vi "Intake.vi"(10 "Enum":enum16{"Retract", "Extend"}(ring)) -> ()   [LabVIEW 2019]
uses:
  <vilib>/Rock Robotics/WPI/ThirdParty/Phoenix-LabVIEW/Motor Controller/Controls/CTRE_Phoenix_MotorControl_ControlMode.ctl
  <vilib>/Rock Robotics/WPI/Solenoid/WPI_SolenoidValue.ctl
  max2020/RoboRIO/Global Data.vi
  max2020/RoboRIO/Refnums.vi
  <vilib>/Rock Robotics/WPI/Solenoid/WPI_SolenoidSetEnum.vi
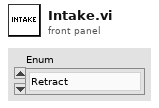
[diagram p1: front panel]
types:
  T1 = typedef "CTRE_Phoenix_MotorControl_ControlMode.ctl" = u16
  T2 = typedef "WPI_RobotDriveDevRef.ctl" = cluster{"DevStatus":errorcluster, "Motors[]":T3[], "Square Inputs":bool, "Max Output":dbl}
  T3 = typedef "WPI_MotorControlDeviceRef.ctl" = cluster{"DeviceStatus":errorcluster, "Type":T4, "PWM":cluster{"PWM Channel":T5, "DeadBand":T6}, "CAN":cluster{"Device Number":u8, "SetOutput VI Ref":variant, "GetOutput VI Ref":variant, "Enable VI Ref":variant, "Disable VI Ref":variant, "Data":variant}, "Invert":bool, "DIO PWM":cluster{"PWM \"Enable\" Channel":T5, "DIOChannel":T7, "PWM Rate":dbl}}
  T4 = typedef "WPI_MotorControlType.ctl" = enum16{"PWM", "CAN", "DIO PWM"}
  T5 = typedef "FPGA_DIOPWMChannel.ctl" = enum8{"PWM 0", "PWM 1", "PWM 2", "PWM 3", "PWM 4", "PWM 5", "PWM 6", "PWM 7", "PWM 8", "PWM 9", "PWM MXP 0", "PWM MXP 1", "PWM MXP 2", "PWM MXP 3", "PWM MXP 4", "PWM MXP 5", "PWM MXP 6", "PWM MXP 7", "PWM MXP 8", "PWM MXP 9", "Invalid"}
  T6 = typedef "WPI_PWMDeadband.ctl" = cluster{"Name":string, "maxPositivePwm":i32, "minPositivePwm":i32, "centerPwm":i32, "maxNegativePwm":i32, "minNegativePwm":i32, "angularRange":u16}
  T7 = typedef "FPGA_DIOChannel.ctl" = enum8{"DIO 0", "DIO 1", "DIO 2", "DIO 3", "DIO 4", "DIO 5", "DIO 6", "DIO 7", "DIO 8", "DIO 9", "DIO MXP 0", "DIO MXP 1", "DIO MXP 2", "DIO MXP 3", "DIO MXP 4", "DIO MXP 5", "DIO MXP 6", "DIO MXP 7", "DIO MXP 8", "DIO MXP 9", "DIO MXP 10", "DIO MXP 11", "DIO MXP 12", "DIO MXP 13", "DIO MXP 14", "DIO MXP 15", "SPI Port CS1", "SPI Port CS2", "SPI Port CS3", "SPI Port MISO", "SPI Port MOSI", "Invalid"}
  T8 = cluster{"ROBOT_DRIVE":T2, "RIGHT_DRIVE":T3, "LEFT_DRIVE":T3, "TURRET":T3, "SHOOTER_MASTER":T3, "HOPPER":T3, "INDEXER":T3, "INTAKE":T3, "CLIMBER_WINCH":T3, "CLIMBER_ARM":T3, "SHOOTER_ANGLE":T3, "SHOOTER_SLAVE":T3, "AGITATOR":T3, "AGITATOR OLD":T3}
  T9 = typedef "WPI_SolenoidDevRef.ctl" = cluster{"DevStatus":errorcluster, "Pneumatics Control Module":u8, "Forward Solenoid Channel":T10, "Reverse Solenoid Channel":T10}
  T10 = typedef "WPI_SolenoidChannel.ctl" = enum8{"Solenoid 0", "Solenoid 1", "Solenoid 2", "Solenoid 3", "Solenoid 4", "Solenoid 5", "Solenoid 6", "Solenoid 7", "Invalid"}
  T11 = typedef "WPI_SolenoidValue.ctl" = enum16{"Off", "On", "Forward", "Reverse"}
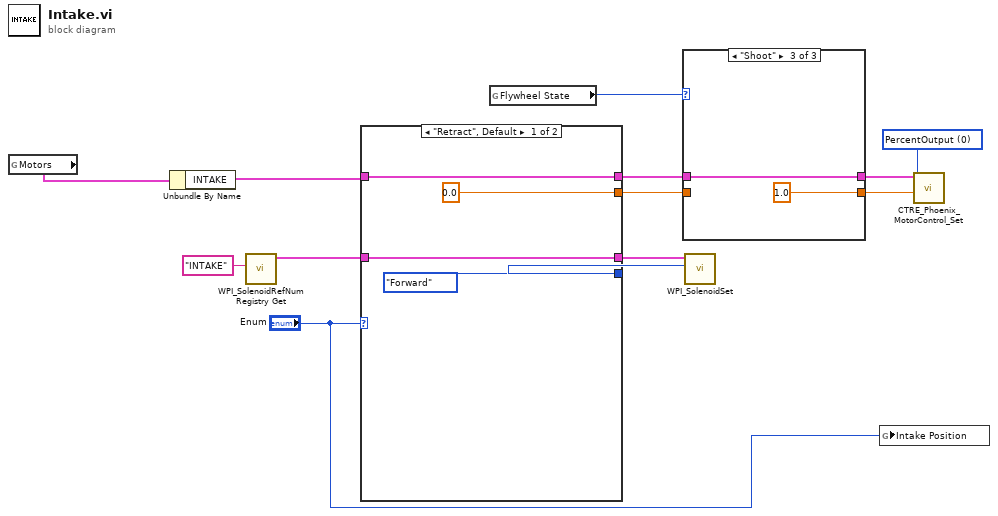
[diagram p0: block diagram]
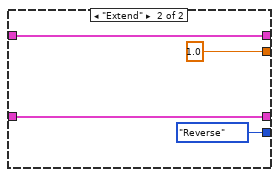
[diagram p4: hidden frame]
diagram:
  w11 = T1 0 items=["PercentOutput"=0, "Position"=1, "Velocity"=2, "Current"=3, "Follower"=5, "MotionProfile"=6, "MotionMagic"=7, "MotionProfileArc"=10, "Disabled"=15] ("Control Mode")
  n1 = global read "Refnums.vi" "Motors"() -> (w13:T8)
  n2 = Unbundle By Name(w13) -> ("INTAKE"=w12:T3)
  n3 = call <vilib>:"WPI_SolenoidRefNum Registry Get.vi"("refnum name"="INTAKE") -> ("SolenoidDevRef"=w9:T9)  [unwired: 9 in, 1 out]
  n4 = case shown="\"Retract\", Default" "Enum" {
    tunnel: w9 -> [w16 w20]
    tunnel: w12 -> [w15 w21]
    tunnel: [WPI_SolenoidValue."Forward" ("Value") WPI_SolenoidValue."Reverse" ("Value")] -> w3
    tunnel: [w15 w21] -> w6
    tunnel: [w16 w20] -> w4
    tunnel: [0.0 ("Output") 1.0 ("Output")] -> w2
    frame "Retract", Default {
    }
    frame "Extend" {
    }
  }
  n5 = global read "Global Data.vi" "Flywheel State"() -> (w8:enum16{"Spin-Up", "Shoot", "Stop"})
  n6 = case shown="\"Shoot\"" w8 {
    tunnel: [w23 w24 1.0] -> w7
    tunnel: w6 -> [w22 w25 w27]
    tunnel: [w22 w25 w27] -> w5
    tunnel: w2 -> [w23 w24 _]
    frame "Spin-Up", Default {
    }
    frame "Stop" {
    }
    frame "Shoot" {
    }
  }
  n7 = call-poly <vilib>:"WPI_SolenoidSet.vi"("Value"=w3, "SolenoidDevRef"=w4) -> ()  [unwired: 8 in, 2 out]
  n8 = global write "Global Data.vi" "Intake Position"("Enum") -> ()
  n9 = call <vilib>:"CTRE_Phoenix_MotorControl_Set.vi"("Output"=w7, "Control Mode"=w11, "PhoenixMotorControlDevRef"=w5) -> ()  [unwired: 7 in, 2 out]
